vi "Read Text Refnum.vi"(8 "error in (no error)":errorcluster, 11 "Text field in":refnum<class "Text field.lvclass">) -> (0 "error out":errorcluster, 2 "Str Refnum":refnum<vi>, 3 "Text field out":refnum<class "Text field.lvclass">)   [LabVIEW 2020, in "Text field.lvclass"]
uses:
  Text field.lvclass
  C:/Users/User/Desktop/Raman Program/Database OOP/source/Field/Field.lvclass
  Field/Field.lvclass/Field.ctl
  Field/Field.lvclass
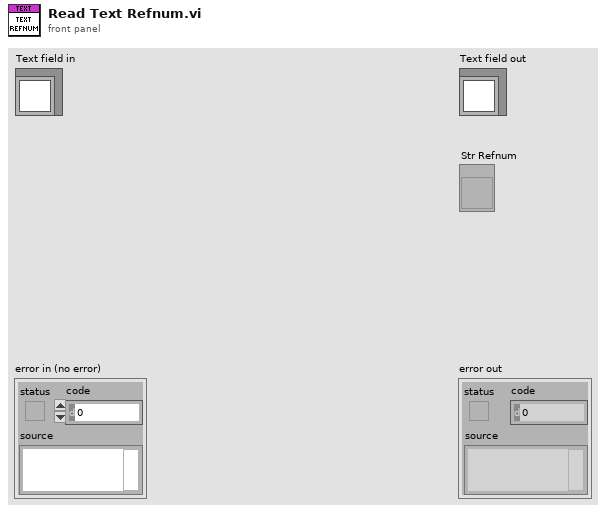
[diagram p1: front panel]
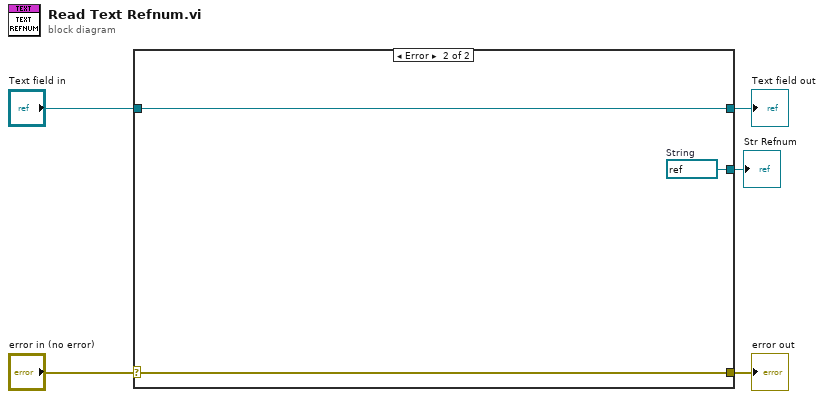
[diagram p0: block diagram]
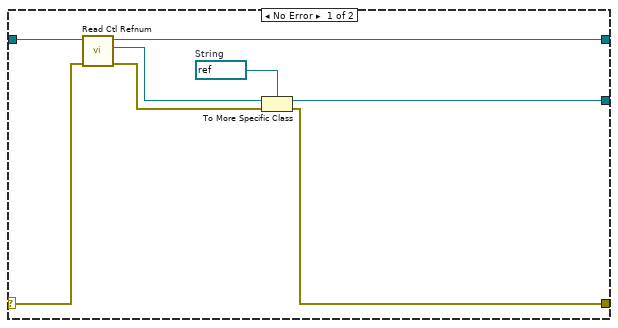
[diagram p2: hidden frame]
diagram:
  n1 = case shown="Error" "error in (no error)" {
    selector: "error in (no error)" -> [w8 w16]
    tunnel: [w6 w16] -> w4
    tunnel: [w12 w15] -> w2
    tunnel: "Text field in" -> [w13 w15]
    tunnel: [w9 w14] -> w1
    frame No Error {
      w10 = refnum<vi> refnum  # String
      n2 = call "Read Ctl Refnum.vi"("error in (no error)"=w8, "Field in"=w13) -> ("error out"=w7:errorcluster, "Ctl Refnum"=w11:refnum<vi>, "Field out"=w12:refnum<class "Text field.lvclass">)  [unwired: 7 in]
      n3 = To More Specific Class(target class=w10, reference=w11, error in=w7) -> (specific class reference=w9:refnum<vi>, error out=w6:errorcluster)
    }
    frame Error {
      w14 = refnum<vi> refnum  # String
    }
  }
  "error out" <- w4
  "Text field out" <- w2
  "Str Refnum" <- w1
